vi "LWXPS_GetVelParams.vi"(0 "XPS Reference IN":refnum<k24>, 5 "LabVIEW error IN":errorcluster) -> (14 "XPS Reference OUT":refnum<k24>, 15 "Returned error code":i32, 16 "Velocity X":dbl, 17 "Velocity Y":dbl, 18 "XPS Error String":string, 19 "LabVIEW error OUT":errorcluster)   [LabVIEW 2014]
uses:
  D:/XPSQ8_LabView_Library/Development/Source/Dll/Newport.XPS.CommandInterface.dll
  Dll/Newport.XPS.CommandInterface.dll
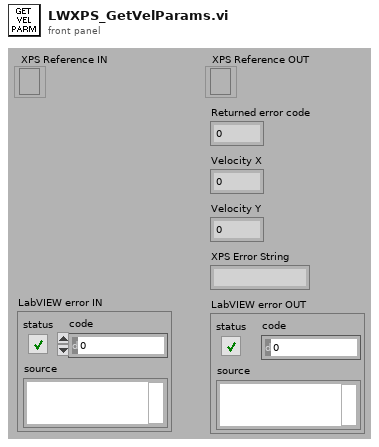
[diagram p1: front panel]
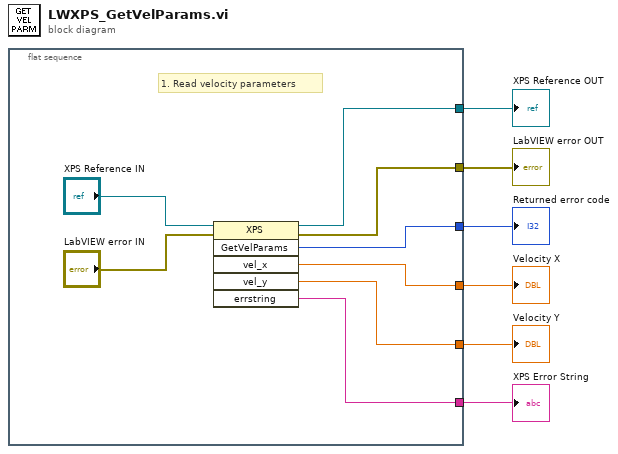
[diagram p0: block diagram]
diagram:
  n1 = flat-sequence {
    tunnel: [w8] -> w6
    tunnel: [w13] -> w5
    tunnel: [w11] -> w4
    tunnel: [w10] -> w1
    tunnel: [w9] -> w3
    tunnel: [w7] -> w2
    frame #0 {
      # "1. Read velocity parameters"
      n2 = invoke class="XPS" method="GetVelParams"(reference="XPS Reference IN", error in="LabVIEW error IN") -> (reference out=w8:refnum<k24>, error out=w13:errorcluster, "GetVelParams"=w11:i32, "vel_x"=w7:dbl, "vel_y"=w10:dbl, "errstring"=w9:string)  [unwired: 4 in]
    }
  }
  "XPS Reference OUT" <- w6
  "LabVIEW error OUT" <- w5
  "Returned error code" <- w4
  "XPS Error String" <- w3
  "Velocity X" <- w2
  "Velocity Y" <- w1
